vi "Module Loop.vi"(8 "error in (no error)":errorcluster, 11 "Volatus Core in":refnum<class "Volatus Core.lvclass">) -> (0 "error out":errorcluster, 3 "Volatus Core out":refnum<class "Volatus Core.lvclass">)   [LabVIEW 2023, in "Volatus.lvlib" / "Volatus Core.lvclass"]
uses:
  Volatus Core.lvclass
  Module/Module.lvclass/Module.ctl
  MessageQ/MessageQ.lvclass/MessageQ.ctl
  Module/Module.lvclass
  Volatus Core.lvclass/Volatus Core.ctl
  Module/Module Status Update.ctl
  MessageQ/MessageQ.lvclass
  Module/State.ctl
  Module Substatus.ctl
  Metric Update.ctl
  StatusTreeValue/StatusTreeValue.lvclass/StatusTreeValue.ctl
  Top Level Module.ctl
  VolatusConfig/VolatusConfigElement/VolatusConfigElement.lvclass
  Reload Options.ctl
  Config Updater/Config Updater.lvclass
  Reload State.ctl
  9d4fff2c-248e-4631-b810-be489ece7d6f.vi
  MessageQ/Delayed Send.vi
  lv-promises/Promises/Promise/Promise.lvclass
  StatusTreeValue/StatusTreeValue.lvclass
  Volatus.lvlib
  C:/dev/volatus/mts-volatus-super/libs/lv-volatus/Volatus/Module/Module.lvclass
  C:/dev/volatus/mts-volatus-super/libs/lv-volatus/Volatus/Volatus Core/Volatus Core.lvclass
panel:
  in  "Events":bool
  in  "Reload Config":bool
  in  "Test Error":bool
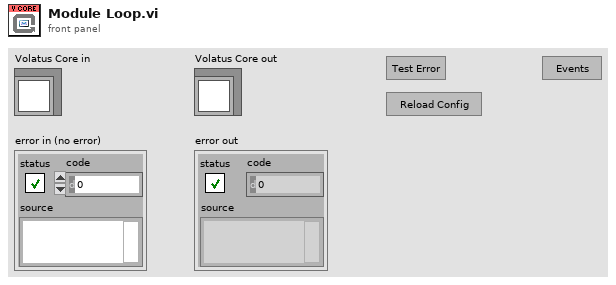
[diagram p1: front panel]
types:
  T1 = enum32{"Invalid", "Standard", "Closed", "Hidden", "Minimized", "Maximized"}
  T2 = typedef "Volatus.lvlib/Module Status Update.ctl" = cluster{"MessageQ":refnum<class "MessageQ.lvclass">, "State":T3, "Hierarchy":string[], "Forwarded":bool}
  T3 = typedef "Volatus.lvlib/Module.lvclass/State.ctl" = enum16{"Unknown", "Launched", "Starting", "Running", "Stopping", "Stopped", "Error - Starting", "Error - Run", "Error - Stopping"}
  T4 = typedef "Volatus.lvlib/Module Substatus.ctl" = cluster{"Hierarchy":string[], "Name":string, "Status":string}
  T5 = typedef "Volatus.lvlib/Metric Update.ctl" = cluster{"Hierarchy":string[], "Name":string, "Value":dbl}
  T6 = typedef "Volatus.lvlib/Volatus Core.lvclass/Top Level Module.ctl" = cluster{"Module":refnum<class "Module.lvclass">, "Config Element":refnum<class "VolatusConfigElement.lvclass">}
  T7 = typedef "Volatus.lvlib/Reload Options.ctl" = cluster{"Updater":refnum<class "Config Updater.lvclass">}
  T8 = typedef "Volatus.lvlib/Volatus Core.lvclass/Reload State.ctl" = enum16{"None", "Stop Modules", "Close Vecto", "Reload", "Restart"}
  T9 = typedef "Volatus.lvlib/Module Status.ctl" = cluster{"Hierarchy":string[], "State":T3, "Substatus":map{string, string}, "Metrics":map{string, dbl}}
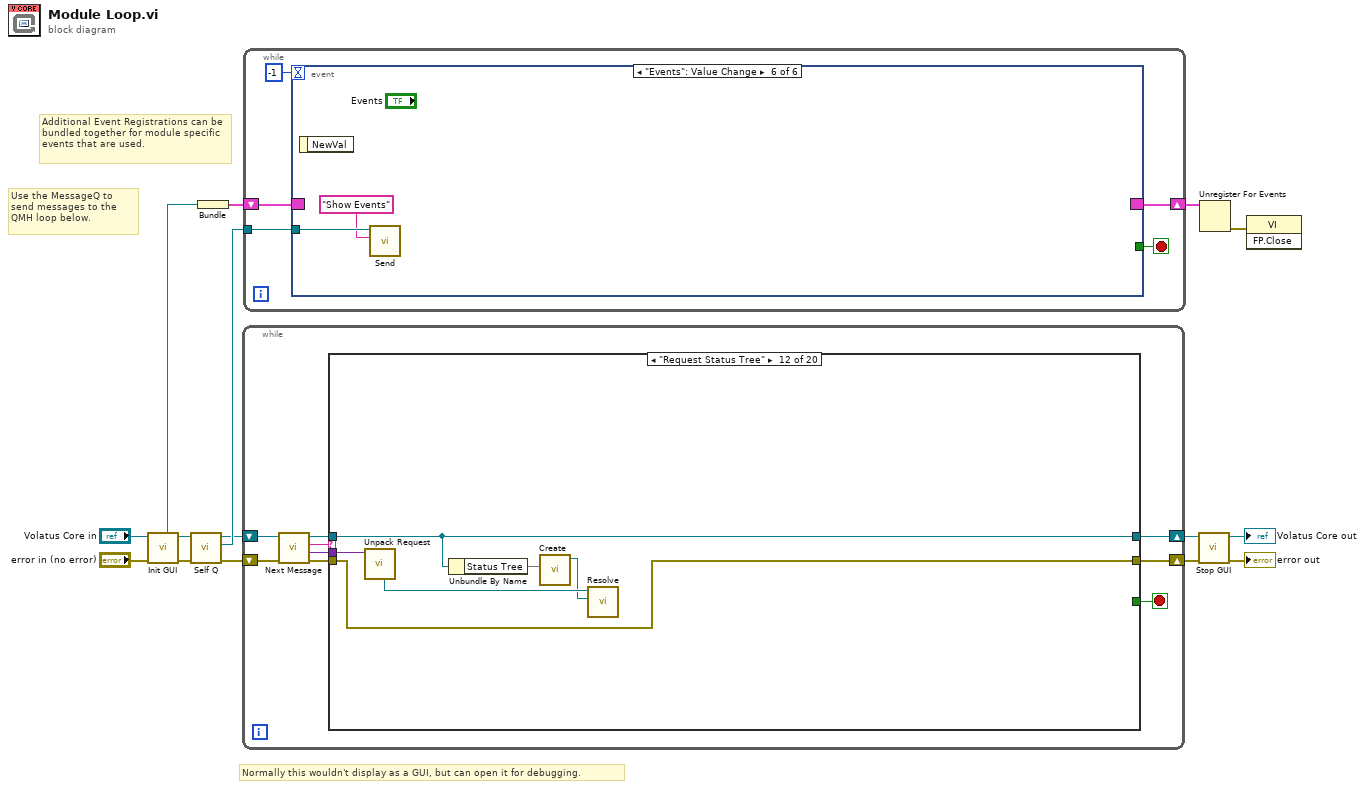
[diagram p0: block diagram]
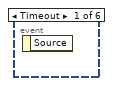
[diagram p2: hidden frame]
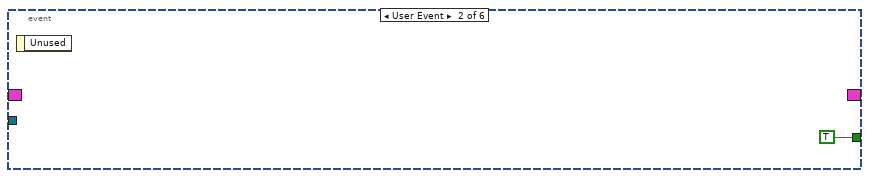
[diagram p3: hidden frame]
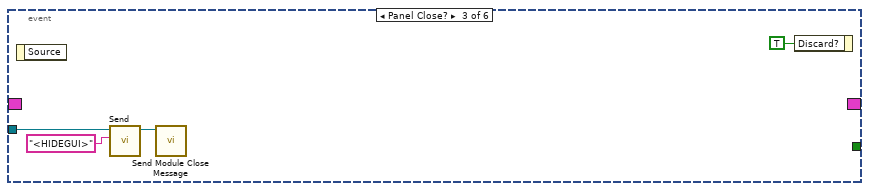
[diagram p4: hidden frame]
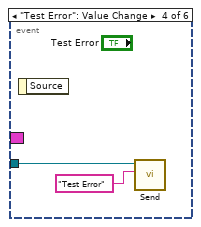
[diagram p5: hidden frame]
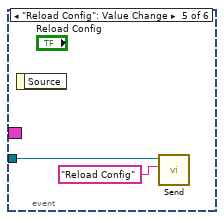
[diagram p6: hidden frame]
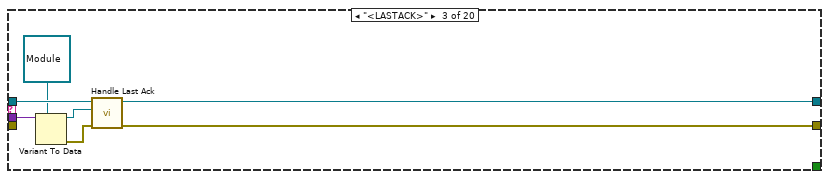
[diagram p9: hidden frame]
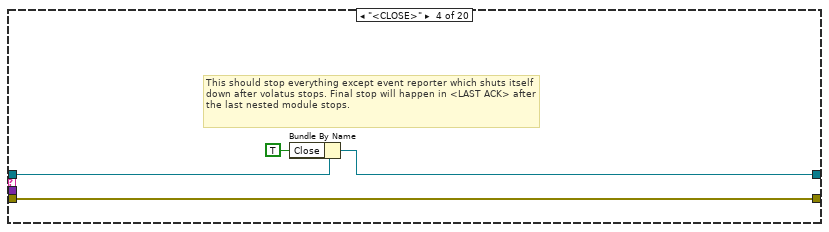
[diagram p10: hidden frame]
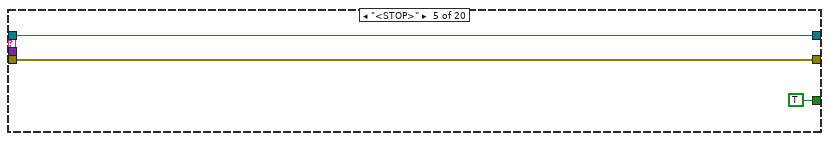
[diagram p11: hidden frame]
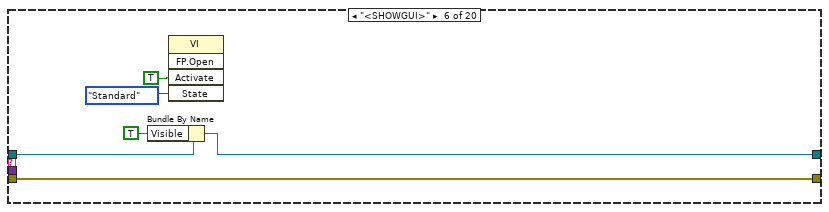
[diagram p12: hidden frame]
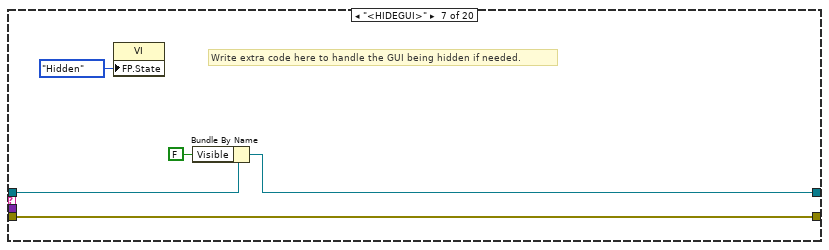
[diagram p13: hidden frame]
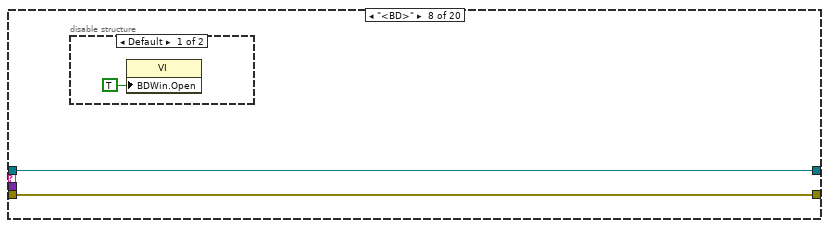
[diagram p14: hidden frame]
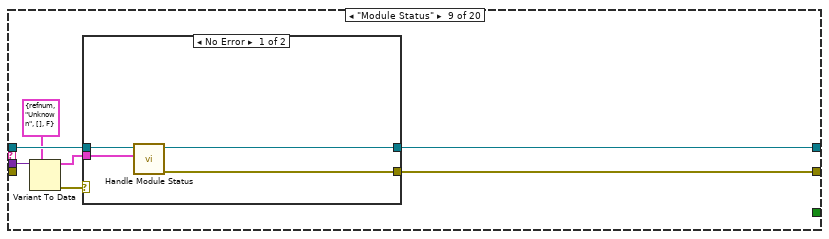
[diagram p16: hidden frame]
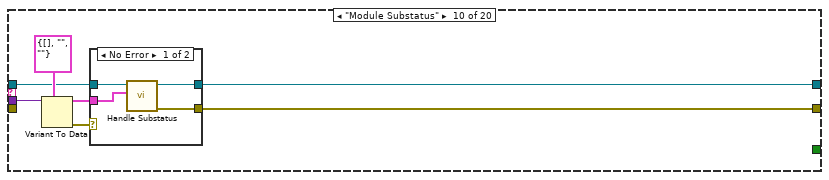
[diagram p18: hidden frame]
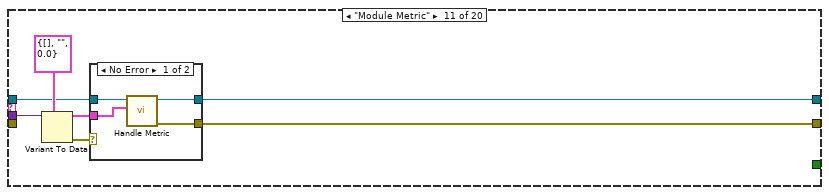
[diagram p20: hidden frame]
diagram:
  # "Normally this wouldn't display as a GUI, but can open it for debugging."
  # "Additional Event Registrations can be bundled together for module specific events that are used."
  # "Use the MessageQ to send messages to the QMH loop below."
  n1 = call "Init GUI.vi"("Module in"="Volatus Core in") -> ("Module out"=w8:refnum<class "Volatus Core.lvclass">, "Event Reg"=w13:refnum<event-registration>)  [unwired: 9 in]
  n2 = call "Self Q.vi"("Module in"=w8) -> ("Self Q"=w7:refnum<class "MessageQ.lvclass">, "Module out"=w6:refnum<class "Volatus Core.lvclass">)  [unwired: 9 in]
  n3 = Bundle("Event Reg"=w13) -> (w9:cluster{"Event Reg":refnum<event-registration>})  [unwired: 1 in]
  n4 = while {
    shift-right: [w17] -> w11
    shift-left: w6 -> [w22]
    shift-right: [w16] -> w12
    shift-left: "error in (no error)" -> [w21]
    stop <- w15 stop-if-true
    n5 = call "Next Message.vi"("error in (no error)"=w21, "Module in"=w22) -> ("error out"=w20:errorcluster, "Data"=w14:variant, "ID"=w19:string, "Module out"=w18:refnum<class "Volatus Core.lvclass">)  [unwired: 6 in]
    n6 = case shown="\"Request Status Tree\"" w19 {
      tunnel: w20 -> [w23 w25 _ w37 w39 w45 w50 w52 _ _ _ w94 _ _ _ _ _ w160 w164 w168]
      tunnel: w18 -> [w24 w26 w33 w36 w40 w46 w51 w53 w61 w71 w84 w98 w103 w119 w125 w141 w146 w157 w162 w169]
      tunnel: [w24 w26 w32 w35 w40 w42 w48 w53 w58 w69 w82 w98 w104 w117 w124 w143 w146 w149 w161 w169] -> w17
      tunnel: [w23 w25 w31 w37 w39 w45 w50 w52 w56 w70 w83 w94 w100 w118 w126 w133 w144 w151 w163 w167] -> w16
      tunnel: [_ _ _ _ TRUE ("Close") _ _ _ _ _ _ _ _ _ _ _ _ _ _ _] -> w15
      tunnel: w14 -> [_ _ w30 _ _ _ _ _ w60 w74 w87 w99 w107 w115 w123 _ _ _ _ _]
      frame Default {
      }
      frame "<TIMEOUT>" {
        # "No message for this module was received in time"
      }
      frame "<LASTACK>" {
        n7 = Variant To Data(type=refnum<class "Module.lvclass"> refnum ("Volatus:Module"), Variant=w30) -> (data=w28:refnum<class "Module.lvclass">, error out=w27:errorcluster)  [unwired: 1 in]
        n8 = call "Handle Last Ack.vi"("error in (no error)"=w27, "Volatus:Module"=w28, "Volatus Core in"=w33) -> ("error out"=w31:errorcluster, "Volatus Core out"=w32:refnum<class "Volatus Core.lvclass">)  [unwired: 7 in]
      }
      frame "<CLOSE>" {
        # "This should stop everything except event reporter which shuts itself down after volatus stops. Final stop will happen in <LAST ACK> after the last nested module stops."
        n9 = Bundle By Name(cluster=w36, "Close"=TRUE) -> (w35:refnum<class "Volatus Core.lvclass">)
      }
      frame "<STOP>" {
      }
      frame "<SHOWGUI>" {
        n10 = Bundle By Name(cluster=w46, "Visible"=TRUE) -> (w42:refnum<class "Volatus Core.lvclass">)
        n11 = invoke class="VI" method="FP.Open"("Activate"=TRUE ("Activate?"), "State"=T1."Standard") -> ()  [unwired: 3 in, 5 out]
      }
      frame "<HIDEGUI>" {
        # "Write extra code here to handle the GUI being hidden if needed."
        n12 = property class="VI"("FP.State"=T1."Hidden" ("Front Panel Window:State")) -> ()  [unwired: 2 in, 2 out]
        n13 = Bundle By Name(cluster=w51, "Visible"=FALSE) -> (w48:refnum<class "Volatus Core.lvclass">)
      }
      frame "<BD>" {
        n14 = disable-structure shown="Default" {
          frame condition #0 (active) {
            n15 = property class="VI"("BDWin.Open"=TRUE ("Block Diagram Window:Open")) -> ()  [unwired: 2 in, 2 out]
          }
          frame condition #1 {
          }
        }
      }
      frame "Module Status" {
        n16 = Variant To Data(type=T2 {"MessageQ"=refnum, "State"=enum."Unknown", "Hierarchy"=[], "Forwarded"=FALSE} ("Module Status"), Variant=w60) -> (data=w57:T2, error out=w55:errorcluster)  [unwired: 1 in]
        n17 = case shown="No Error" w55 {
          selector: w55 -> [_ w67]
          tunnel: w61 -> [w64 w66]
          tunnel: [w63 w66] -> w58
          tunnel: w57 -> [w65 _]
          tunnel: [w62 w67] -> w56
          frame No Error {
            n18 = call "Handle Module Status.vi"("Module Status"=w65, "Volatus Core in"=w64) -> ("error out"=w62:errorcluster, "Volatus Core out"=w63:refnum<class "Volatus Core.lvclass">)  [unwired: 8 in]
          }
          frame Error {
          }
        }
      }
      frame "Module Substatus" {
        n19 = Variant To Data(type=T4 {"Hierarchy"=[], "Name"="", "Status"=""} ("Module Substatus"), Variant=w74) -> (data=w68:T4, error out=w72:errorcluster)  [unwired: 1 in]
        n20 = case shown="No Error" w72 {
          selector: w72 -> [_ w80]
          tunnel: w71 -> [w78 w79]
          tunnel: [w75 w80] -> w70
          tunnel: [w76 w79] -> w69
          tunnel: w68 -> [w77 _]
          frame No Error {
            n21 = call "Handle Substatus.vi"("Module Substatus"=w77, "Volatus Core in"=w78) -> ("error out"=w75:errorcluster, "Volatus Core out"=w76:refnum<class "Volatus Core.lvclass">)  [unwired: 8 in]
          }
          frame Error {
          }
        }
      }
      frame "Module Metric" {
        n22 = Variant To Data(type=T5 {"Hierarchy"=[], "Name"="", "Value"=0.0} ("Metric Update"), Variant=w87) -> (data=w81:T5, error out=w85:errorcluster)  [unwired: 1 in]
        n23 = case shown="No Error" w85 {
          selector: w85 -> [_ w93]
          tunnel: w84 -> [w91 w92]
          tunnel: [w88 w93] -> w83
          tunnel: [w89 w92] -> w82
          tunnel: w81 -> [w90 _]
          frame No Error {
            n24 = call "Handle Metric.vi"("Metric Update"=w90, "Volatus Core in"=w91) -> ("error out"=w88:errorcluster, "Volatus Core out"=w89:refnum<class "Volatus Core.lvclass">)  [unwired: 8 in]
          }
          frame Error {
          }
        }
      }
      frame "Request Status Tree" {
        n25 = call "Unpack Request.vi"("Request Data"=w99) -> ("Promise"=w96:refnum<class "Promise.lvclass">)  [unwired: 8 in, 2 out]
        n26 = Unbundle By Name(w98) -> ("Status Tree"=w97:map{string[], T9})
        n27 = call "Create.vi"("Status Tree"=w97) -> ("StatusTreeValue out"=w95:refnum<class "StatusTreeValue.lvclass">)  [unwired: 10 in]
        n28 = call "Resolve.vi"("Result (None)"=w95, "Promise in"=w96) -> ()  [unwired: 8 in, 2 out]
      }
      frame "Launch Module" {
        n29 = Variant To Data(type=T6 {"Module"=refnum, "Config Element"=refnum} ("Top Level Module"), Variant=w107) -> (data=w105:T6, error out=w108:errorcluster)  [unwired: 1 in]
        n30 = Unbundle By Name(w105) -> ("Module"=w102:refnum<class "Module.lvclass">, "Config Element"=w101:refnum<class "VolatusConfigElement.lvclass">)
        n31 = call "Launch Nested.vi"("error in (no error)"=w108, "Config Element"=w101, "Nested Module"=w102, "Parent in"=w103) -> ("error out"=w100:errorcluster, "Parent out"=w104:refnum<class "Volatus Core.lvclass">)  [unwired: 5 in, 1 out]
      }
      frame "New Config" {
        n32 = Variant To Data(type=path "", Variant=w115) -> (data=w112:path, error out=w114:errorcluster)  [unwired: 1 in]
        n33 = call "Read Volatus INI.vi"("error in (no error)"=w114, "INI Path (Default)"=w112, "Volatus Core in"=w119) -> ("error out"=w120:errorcluster, "Volatus Core out"=w110:refnum<class "Volatus Core.lvclass">)  [unwired: 7 in]
        n34 = call "Send Hide GUI Message.vi"("error in (no error)"=w120, "Module in"=w110) -> ("error out"=w111:errorcluster, "Module out"=w109:refnum<class "Volatus Core.lvclass">)  [unwired: 8 in]
        n35 = call "Send to Self.vi"("error in (no error)"=w111, "Message ID"="Reload Config", "Module in"=w109) -> ("error out"=w118:errorcluster, "Module out"=w117:refnum<class "Volatus Core.lvclass">)  [unwired: 7 in]
      }
      frame "Reload Config" {
        # "Ignoring errors, defaults are default if sender doesn't specify options."
        n36 = Variant To Data(type=T7 {"Updater"=refnum} ("Reload Options"), Variant=w123) -> (data=w121:T7)  [unwired: 1 in, 1 out]
        n37 = call "Prepare Config Reload.vi"("Reload Options"=w121, "Volatus Core in"=w125) -> ("error out"=w126:errorcluster, "Volatus Core out"=w124:refnum<class "Volatus Core.lvclass">)  [unwired: 8 in]
      }
      frame "Close Vecto" {
        # "Need to give some time for async components in Vecto to wrap up. Eventually I should make vecto shutdown more deterministic."
        n38 = call "Update Splash Status.vi"("Status"="Closing Vecto", "Volatus Core in"=w141) -> ("Volatus Core out"=w128:refnum<class "Volatus Core.lvclass">)  [unwired: 8 in, 1 out]
        n39 = call "Close Vecto.vi"("Volatus Core in"=w128) -> ("error out"=w134:errorcluster, "Volatus Core out"=w138:refnum<class "Volatus Core.lvclass">)  [unwired: 9 in]
        n40 = call "Stall Data Flow.vim"("value in"=w138, "milliseconds to wait"=u32 2000) -> ("value out"=w130:refnum<class "Volatus Core.lvclass">)  [unwired: 1 out]
        n41 = call "Try Update Config.vi"("Volatus Core in"=w130) -> ("error out"=w135:errorcluster, "Volatus Core out"=w137:refnum<class "Volatus Core.lvclass">)  [unwired: 9 in]
        n42 = call "Report Event.vi"("Message"="Reloading configuration", "Module in"=w137) -> ("Module out"=w132:refnum<class "Volatus Core.lvclass">)  [unwired: 8 in, 1 out]
        n43 = call "Init Node.vi"("First Launch"=FALSE ("Launch Events"), "Volatus Core in"=w132) -> ("error out"=w136:errorcluster, "Volatus Core out"=w139:refnum<class "Volatus Core.lvclass">)  [unwired: 8 in]
        n44 = Merge Errors(w134, w135, w136) -> (w133:errorcluster)
        n45 = Bundle By Name(cluster=w139, "Reload State"=Reload_State."None") -> (w143:refnum<class "Volatus Core.lvclass">)
      }
      frame "Show Events" {
        n46 = Unbundle By Name(w146) -> ("Event Reporter"=w145:refnum<class "MessageQ.lvclass">)
        n47 = call "Send Show GUI Message.vi"("MessageQ"=w145) -> ("error out"=w144:errorcluster)  [unwired: 10 in]
      }
      frame "Start" {
        n48 = call "Start Vecto.vi"("error in (no error)"=w160, "Volatus Core in"=w157) -> ("error out"=w159:errorcluster, "Volatus Core out"=w155:refnum<class "Volatus Core.lvclass">)  [unwired: 8 in]
        n49 = call "Launch Config Module.vi"("error in (no error)"=w159, "Volatus Core in"=w155) -> ("error out"=w156:errorcluster, "Volatus Core out"=w153:refnum<class "Volatus Core.lvclass">)  [unwired: 8 in]
        n50 = call "Launch HW Info.vi"("error in (no error)"=w156, "Volatus Core in"=w153) -> ("error out"=w154:errorcluster, "Volatus Core out"=w152:refnum<class "Volatus Core.lvclass">)  [unwired: 8 in]
        n51 = call "Launch Configured Tasks.vi"("error in (no error)"=w154, "Volatus Core in"=w152) -> ("error out"=w158:errorcluster, "Volatus Core out"=w150:refnum<class "Volatus Core.lvclass">)  [unwired: 8 in]
        n52 = call "Delayed Send to Self.vi"("Delay ms"=2000, "error in (no error)"=w158, "Message ID"="Hide Splash", "Module in"=w150) -> ("error out"=w151:errorcluster, "Module out"=w149:refnum<class "Volatus Core.lvclass">)  [unwired: 6 in]
      }
      frame "Hide Splash" {
        n53 = call "Hide Splash.vi"("error in (no error)"=w164, "Volatus Core in"=w162) -> ("error out"=w163:errorcluster, "Volatus Core out"=w161:refnum<class "Volatus Core.lvclass">)  [unwired: 8 in]
      }
      frame "Test Error" {
        n54 = call <vilib>:"Error Cluster From Error Code.vi"("error in (no error)"=w168, "error message (\"\")"="Error generated for testing module error reporting.", "error code (0)"=1) -> ("error out"=w167:errorcluster)  [unwired: 6 in]
      }
    }
  }
  n55 = while {
    tunnel: w7 -> [w174]
    shift-right: [w172] -> w10
    shift-left: w9 -> [w173]
    stop <- w171 stop-if-true
    n56 = event shown="[5] \"Events\": Value Change" {
      selector: w173 -> [_ _ _ _ _ _]
      dyn-events: [_ _ _ _ _ _] -> w172
      timeout: -1 -> [_ _ _ _ _ _]
      tunnel: w174 -> [_ _ w178 w181 w183 w185]
      tunnel: [_ TRUE _ _ _ _] -> w171
      event Timeout {
        n57 = event-data() -> ()  [unwired: 1 in, 1 out]
      }
      event User Event {
        n58 = event-data() -> ()  [unwired: 1 in, 1 out]
      }
      event Panel Close? {
        n59 = event-data() -> ()  [unwired: 1 in, 1 out]
        n60 = call "Send.vi"("ID"="<HIDEGUI>", "MessageQ in"=w178) -> ("MessageQ out"=w176:refnum<class "MessageQ.lvclass">)  [unwired: 8 in, 1 out]
        n61 = call "Send Module Close Message.vi"("MessageQ"=w176) -> ()  [unwired: 10 in, 1 out]
        n62 = event-data("Discard?"=TRUE) -> ()  [unwired: 1 in, 1 out]
      }
      event "Test Error": Value Change {
        n63 = event-data() -> ()  [unwired: 1 in, 1 out]
        n64 = call "Send.vi"("ID"="Test Error", "MessageQ in"=w181) -> ()  [unwired: 8 in, 2 out]
      }
      event "Reload Config": Value Change {
        n65 = event-data() -> ()  [unwired: 1 in, 1 out]
        n66 = call "Send.vi"("ID"="Reload Config", "MessageQ in"=w183) -> ()  [unwired: 8 in, 2 out]
      }
      event "Events": Value Change {
        n67 = event-data() -> ()  [unwired: 1 in, 1 out]
        n68 = call "Send.vi"("ID"="Show Events", "MessageQ in"=w185) -> ()  [unwired: 8 in, 2 out]
      }
    }
  }
  n69 = call "Stop GUI.vi"("error in (no error)"=w12, "Module in"=w11) -> ("error out"=→"error out":errorcluster, "Module out"=→"Volatus Core out":refnum<class "Volatus Core.lvclass">)  [unwired: 8 in]
  n70 = Unregister For Events(event registration refnum=w10) -> (error out=w1:errorcluster)  [unwired: 1 in]
  n71 = invoke class="VI" method="FP.Close"(error in=w1) -> ()  [unwired: 2 in, 3 out]
